vi "NetworkStreamProcess.vi"(0 "WaveformConfiguration":T1, 11 "error in (no error)":errorcluster) -> ()   [LabVIEW 2017]
uses:
  WaveformAcqModule/module/execution/Export.ctl
  StreamState.ctl
  StreamHeader.ctl
  globals.vi
  WaveformAcqModule/module/execution/WaveformAcq runtime.lvclass
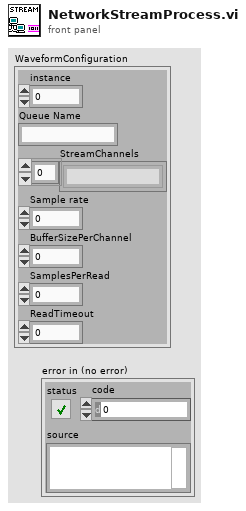
[diagram p1: front panel]
types:
  T1 = typedef "WaveformAcq runtime.lvclass/Export.ctl" = cluster{"instance":i32, "Queue Name":string, "StreamChannels":string[], "Sample rate":i32, "BufferSizePerChannel":i32, "SamplesPerRead":i32, "ReadTimeout":dbl}
  T2 = typedef "StreamHeader.ctl" = cluster{"Channels":string[], "SampleRate":i32}
  T3 = typedef "StreamState.ctl" = enum16{"Idle", "Listening", "Header", "Streaming", "Disconnecting"}
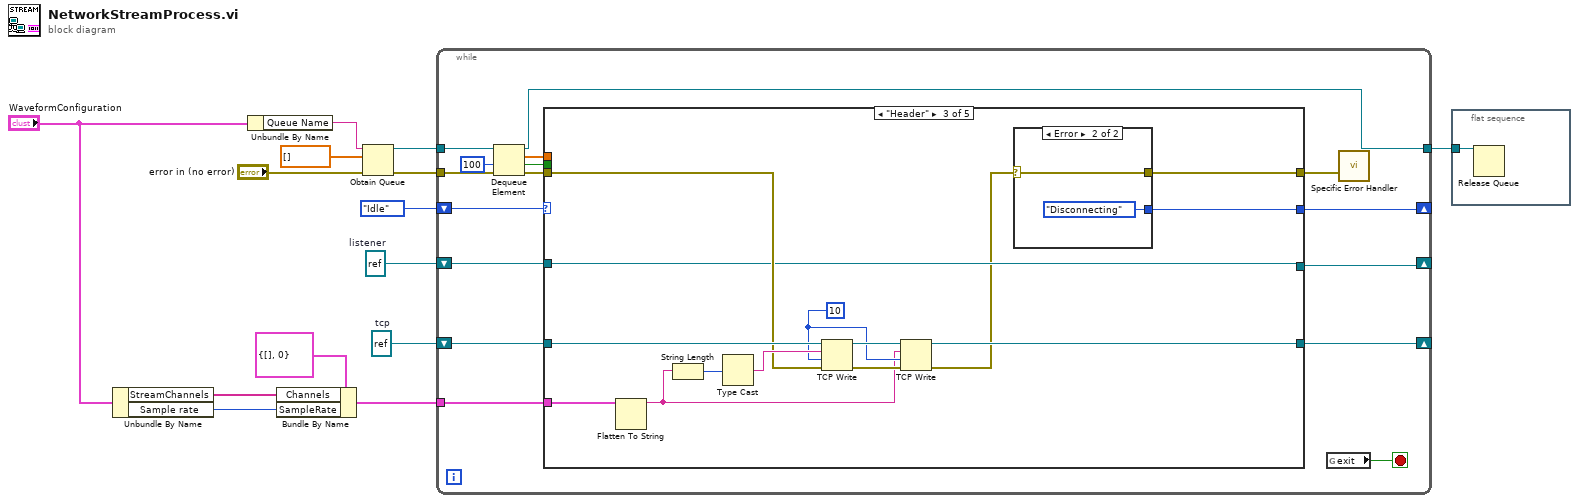
[diagram p0: block diagram]
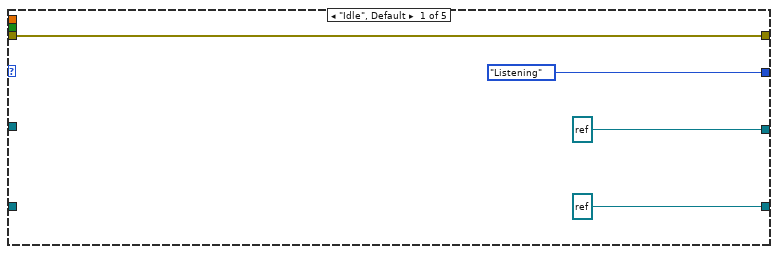
[diagram p2: hidden frame]
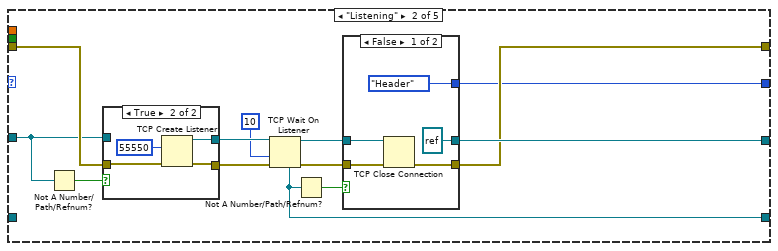
[diagram p3: hidden frame]
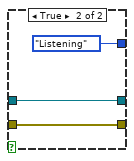
[diagram p4: hidden frame]
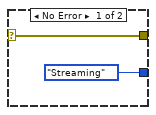
[diagram p6: hidden frame]
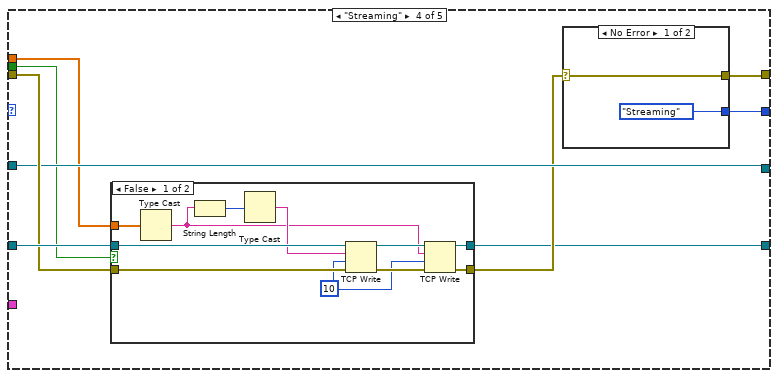
[diagram p7: hidden frame]
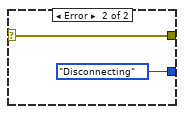
[diagram p8: hidden frame]
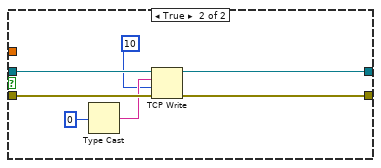
[diagram p9: hidden frame]
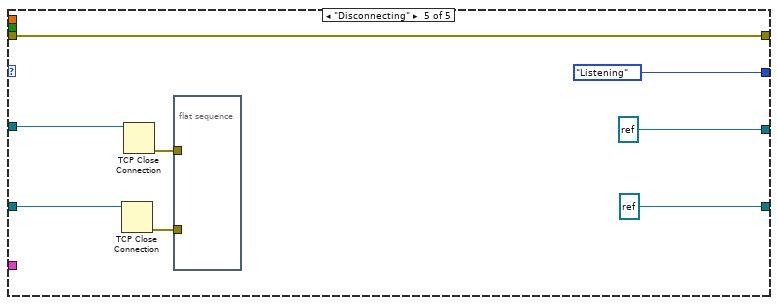
[diagram p10: hidden frame]
diagram:
  w7 = refnum<k5> refnum  # tcp
  w8 = refnum<k5> refnum  # listener
  n1 = Unbundle By Name("WaveformConfiguration") -> ("StreamChannels"=w2:string[], "Sample rate"=w1:i32)
  n2 = Unbundle By Name("WaveformConfiguration") -> ("Queue Name"=w6:string)
  n3 = Bundle By Name(cluster=T2 {"Channels"=[], "SampleRate"=0} ("StreamHeader"), "Channels"=w2, "SampleRate"=w1) -> (w3:T2)
  n4 = Obtain Queue(name (unnamed)=w6, element data type=sgl[] [], error in (no error)="error in (no error)") -> (queue out=w12:refnum<queue>, error out=w13:errorcluster)  [unwired: 2 in, 1 out]
  n5 = while {
    tunnel: w12 -> [w30]
    tunnel: w13 -> [w29]
    tunnel: [w27] -> w14
    shift-right: [w23] -> _
    shift-left: StreamState."Idle" ("StreamState") -> [w25]
    shift-right: [w18] -> _
    shift-left: w8 -> [w21]
    shift-right: [w17] -> _
    shift-left: w7 -> [w16]
    tunnel: w3 -> [w15]
    stop <- w26 stop-if-true
    n6 = Dequeue Element(queue=w30, timeout in ms (-1)=100, error in (no error)=w29) -> (queue out=w27:refnum<queue>, element=w19:sgl[], timed out?=w20:bool, error out=w24:errorcluster)
    n7 = case shown="\"Header\"" w25 {
      tunnel: w24 -> [w31 w46 w72 w87 w111]
      tunnel: [StreamState."Listening" ("StreamState") w35 w68 w86 StreamState."Listening" ("StreamState")] -> w23
      tunnel: [w31 w36 w64 w81 w111] -> w22
      tunnel: w21 -> [_ w45 w66 w85 w118]
      tunnel: w20 -> [_ _ _ w84 _]
      tunnel: w19 -> [_ _ _ w83 _]
      tunnel: [refnum<k5> refnum ("listener ID") w38 w66 w85 refnum<k5> refnum ("listener")] -> w18
      tunnel: [refnum<k5> refnum ("listener ID") w37 w67 w80 refnum<k5> refnum ("tcp")] -> w17
      tunnel: w16 -> [_ _ w75 w88 w117]
      tunnel: w15 -> [_ _ w63 _ _]
      frame "Idle", Default {
      }
      frame "Listening" {
        n8 = Not A Number/Path/Refnum?(number/path/refnum=w45) -> (NaN/Path/Refnum?=w47:bool)
        n9 = case shown="True" w47 {
          tunnel: w46 -> [w56 w60]
          tunnel: [w57 w59] -> w44
          tunnel: w45 -> [w57 _]
          tunnel: [w56 w58] -> w43
          frame False {
          }
          frame True {
            n10 = TCP Create Listener(8:w60, 10:u16 55550 ("port")) -> (0:w58:errorcluster, 3:w59:refnum<k5>)  [unwired: 3 in, 1 out]
          }
        }
        n11 = TCP Wait On Listener(8:w43, 9:10 ("timeout ms (wait forever: -1)"), 11:w44) -> (0:w40:errorcluster, 3:w39:refnum<k5>, 4:w37:refnum<k5>)  [unwired: 1 in, 2 out]
        n12 = Not A Number/Path/Refnum?(number/path/refnum=w37) -> (NaN/Path/Refnum?=w41:bool)
        n13 = case shown="False" w41 {
          tunnel: w40 -> [w51 w54]
          tunnel: w39 -> [w52 w55]
          tunnel: [refnum<k5> refnum ("listener ID") w55] -> w38
          tunnel: [w50 w54] -> w36
          tunnel: [StreamState."Header" ("StreamState") StreamState."Listening" ("StreamState")] -> w35
          frame False {
            n14 = TCP Close Connection(connection ID=w52, error in (no error)=w51) -> (error out=w50:errorcluster)  [unwired: 1 in, 1 out]
          }
          frame True {
          }
        }
      }
      frame "Header" {
        w69 = 10 ("timeout ms (25000)")
        n15 = Flatten To String(anything=w63) -> (data string=w62:string)  [unwired: 3 in, 2 out]
        n16 = String Length(string=w62) -> (length=w74:i32)
        n17 = Type Cast(x=w74) -> (*(type *) &x=w73:string)  [unwired: 1 in]
        n18 = TCP Write(connection ID=w75, data in=w73, error in (no error)=w72, 9:w69) -> (connection ID out=w71:refnum<k5>, error out=w70:errorcluster)  [unwired: 1 out]
        n19 = TCP Write(connection ID=w71, data in=w62, error in (no error)=w70, 9:w69) -> (connection ID out=w67:refnum<k5>, error out=w65:errorcluster)  [unwired: 1 out]
        n20 = case shown="Error" w65 {
          selector: w65 -> [w76 w79]
          tunnel: [StreamState."Streaming" ("StreamState") StreamState."Disconnecting" ("StreamState")] -> w68
          tunnel: [w76 w79] -> w64
          frame No Error {
          }
          frame Error {
          }
        }
      }
      frame "Streaming" {
        n21 = case shown="False" w84 {
          tunnel: w88 -> [w103 w110]
          tunnel: w87 -> [w100 w109]
          tunnel: [w96 w108] -> w82
          tunnel: [w95 w107] -> w80
          tunnel: w83 -> [w94 _]
          frame False {
            w97 = 10 ("timeout ms (25000)")
            n22 = Type Cast(x=w94) -> (*(type *) &x=w93:string)  [unwired: 1 in]
            n23 = String Length(string=w93) -> (length=w102:i32)
            n24 = Type Cast(x=w102) -> (*(type *) &x=w101:string)  [unwired: 1 in]
            n25 = TCP Write(connection ID=w103, data in=w101, error in (no error)=w100, 9:w97) -> (connection ID out=w99:refnum<k5>, error out=w98:errorcluster)  [unwired: 1 out]
            n26 = TCP Write(connection ID=w99, data in=w93, error in (no error)=w98, 9:w97) -> (connection ID out=w95:refnum<k5>, error out=w96:errorcluster)  [unwired: 1 out]
          }
          frame True {
            n27 = Type Cast(x=0) -> (*(type *) &x=w105:string)  [unwired: 1 in]
            n28 = TCP Write(connection ID=w110, data in=w105, error in (no error)=w109, 9:10 ("timeout ms (25000)")) -> (connection ID out=w107:refnum<k5>, error out=w108:errorcluster)  [unwired: 1 out]
          }
        }
        n29 = case shown="No Error" w82 {
          selector: w82 -> [w89 w92]
          tunnel: [StreamState."Streaming" ("StreamState") StreamState."Disconnecting" ("StreamState")] -> w86
          tunnel: [w89 w92] -> w81
          frame No Error {
          }
          frame Error {
          }
        }
      }
      frame "Disconnecting" {
        n30 = TCP Close Connection(connection ID=w117) -> (error out=w114:errorcluster)  [unwired: 2 in, 1 out]
        n31 = TCP Close Connection(connection ID=w118) -> (error out=w113:errorcluster)  [unwired: 2 in, 1 out]
        n32 = flat-sequence {
          tunnel: w114 -> [_]
          tunnel: w113 -> [_]
          frame #0 {
          }
        }
      }
    }
    n33 = global read "globals.vi" "exit"() -> (w26:bool)
    n34 = call "Specific Error Handler"("Error to Check"=w22) -> ()  [unwired: 11 in, 4 out]
  }
  n35 = flat-sequence {
    tunnel: w14 -> [w119]
    frame #0 {
      n36 = Release Queue(queue=w119) -> ()  [unwired: 2 in, 3 out]
    }
  }
